vi "Get All Performance Channels.vi"(8 "error in (no error)":errorcluster, 11 "Item Ref in":T1 format="%.0x") -> (0 "error out":errorcluster, 2 "Channels refs":T1[](array[typedef]) format="%.0x", 3 "Item Ref out":T1 format="%.0x")   [LabVIEW 2017, in "DSF Shared.lvlib"]
uses:
  DSF Shared.lvlib
  <vilib>/NI Veristand/Custom Device API/Custom Device Item Ref.ctl
  <vilib>/NI Veristand/Custom Device API/Custom Device API.lvlib
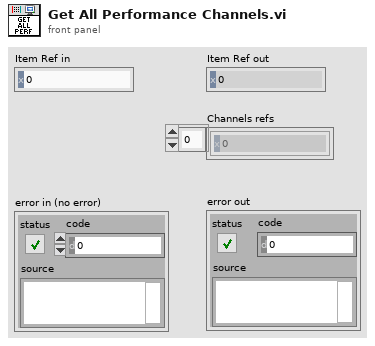
[diagram p1: front panel]
types:
  T1 = typedef "Custom Device API.lvlib/Custom Device Item Ref.ctl" = u64
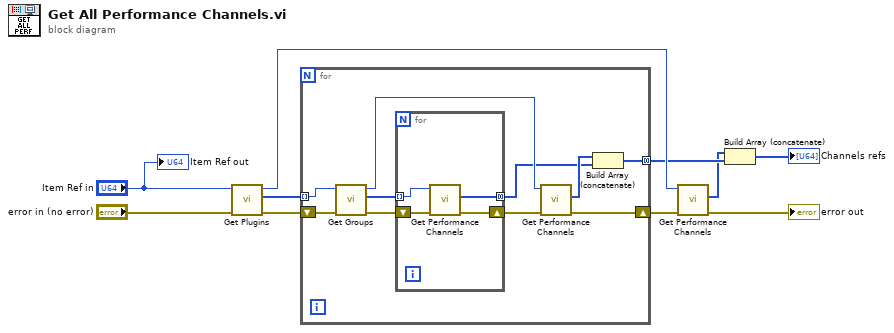
[diagram p0: block diagram]
diagram:
  n1 = call "Get Plugins.vi"("error in (no error)"="error in (no error)", "Item Ref in"="Item Ref in") -> ("error out"=w10:errorcluster, "Plugin refs"=w9:T1[], "Item Ref out"=w7:T1)  [unwired: 7 in]
  n2 = for {
    shift-right: [w15] -> w8
    shift-left: w10 -> [w20]
    tunnel: w9 -> [w19] mode=indexing
    tunnel: [w14] -> w2 mode=concatenating
    n3 = call "Get Groups.vi"("error in (no error)"=w20, "Plugin Ref in"=w19) -> ("error out"=w18:errorcluster, "Group refs"=w17:T1[], "Plugin Ref out"=w13:T1)  [unwired: 7 in]
    n4 = for {
      shift-right: [w22] -> w16
      shift-left: w18 -> [w24]
      tunnel: w17 -> [w23] mode=indexing
      tunnel: [w21] -> w11 mode=concatenating
      n5 = call "Get Performance Channels.vi"("error in (no error)"=w24, "Item Ref in"=w23) -> ("error out"=w22:errorcluster, "Channels refs"=w21:T1[])  [unwired: 7 in, 1 out]
    }
    n6 = call "Get Performance Channels.vi"("error in (no error)"=w16, "Item Ref in"=w13) -> ("error out"=w15:errorcluster, "Channels refs"=w12:T1[])  [unwired: 7 in, 1 out]
    n7 = Build Array (concatenate)(w12, w11) -> (w14:T1[])
  }
  n8 = call "Get Performance Channels.vi"("error in (no error)"=w8, "Item Ref in"=w7) -> ("error out"=→"error out":errorcluster, "Channels refs"=w1:T1[])  [unwired: 7 in, 1 out]
  n9 = Build Array (concatenate)(w1, w2) -> (→"Channels refs":T1[])
  "Item Ref out" <- "Item Ref in"
